vi "FRCts20_WebMethods_Division_PUT.vi"(7 "httpRequestID":u32, 10 "division":string, 11 "competition":string) -> ()   [LabVIEW 2014]
doc: "This method is not implemented."
uses:
  FRCts20_WebMethods.lvlib
  <vilib>/wsapi/NI_WebServices.lvlib
panel:
  in  "query":string
  # "e"
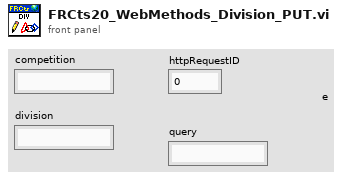
[diagram p1: front panel]
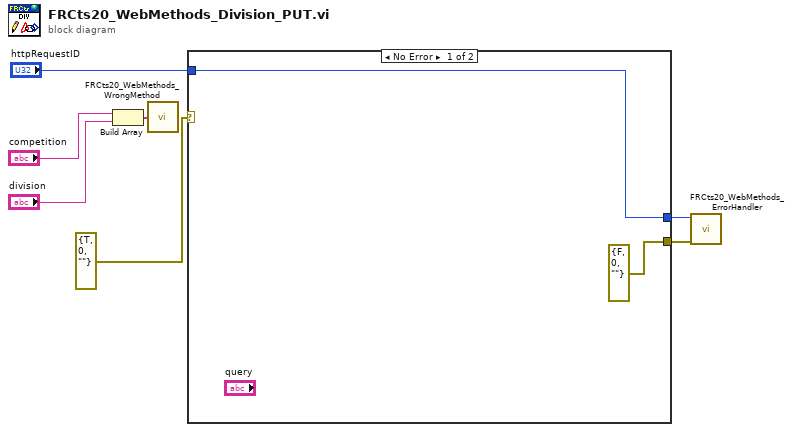
[diagram p0: block diagram]
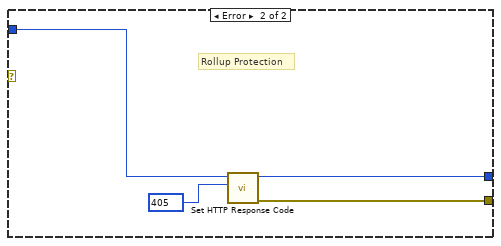
[diagram p2: hidden frame]
diagram:
  n1 = Build Array("competition", "division") -> (w7:string[])
  n2 = call "FRCts20_WebMethods_WrongMethod.vi"(4:w7) -> ()  [unwired: 4 in, 1 out]
  n3 = case shown="No Error" errorcluster {"status"=TRUE, "code"=0, "source"=""} ("error IO") {
    tunnel: "httpRequestID" -> [w8 w13]
    tunnel: [w8 w11] -> w2
    tunnel: [errorcluster {"status"=FALSE, "code"=0, "source"=""} ("error out") w10] -> w3
    frame No Error {
    }
    frame Error {
      w12 = 405 items=["100"=100, "101"=101, "200"=200, "201"=201, "202"=202, "203"=203, "204"=204, "205"=205, "206"=206, "300"=300, "301"=301, "302"=302, "303"=303, "304"=304, "305"=305, "306"=306, "307"=307, "400"=400, "401"=401, "402"=402, "403"=403, "404"=404, "405"=405, "406"=406, "407"=407, "408"=408, "409"=409, "410"=410, "411"=411, "412"=412, "413"=413, "414"=414, "415"=415, "416"=416, "417"=417, "500"=500, "501"=501, "502"=502, "503"=503, "504"=504, "505"=505] ("response code (200)")
      # "Rollup Protection"
      n4 = call <vilib>:"Set HTTP Response Code.vi"("response code (200)"=w12, "httpRequestID"=w13) -> ("error out"=w10:errorcluster, "httpRequestID out"=w11:u32)  [unwired: 8 in]
    }
  }
  n5 = call "FRCts20_WebMethods_ErrorHandler.vi"("error in"=w3, "httpRequestID"=w2) -> ()  [unwired: 9 in, 1 out]
